vi "backup step.vi"(8 "error in (no error)":errorcluster, 10 "page":i32, 11 "backup_ref":u64) -> (0 "error out":errorcluster)   [LabVIEW 2020, in "sqlite3.lvlib"]
uses:
  sqlite3.lvlib
  errstr.vi
  bin/sqlite3_64.dll
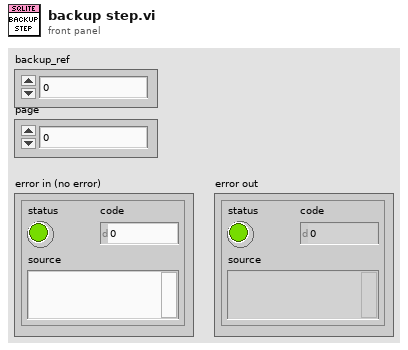
[diagram p1: front panel]
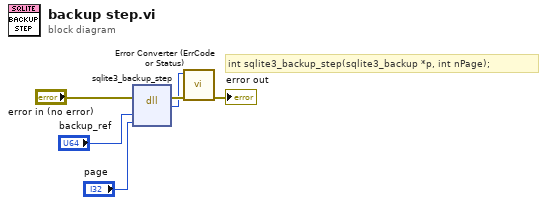
[diagram p0: block diagram]
diagram:
  # "int sqlite3_backup_step(sqlite3_backup *p, int nPage);"
  n1 = dll-call lib="D:/Project/Labview-Projects/database-configuration/externals/sqlite3/Source/bin/sqlite3_*.*" fn="sqlite3_backup_step"(error in="error in (no error)", "backup_ref"="backup_ref", "page"="page") -> (error out=w3:errorcluster, "return type"=w1:i32)  [unwired: 4 in, 1 out]
  n2 = call "Error Converter (ErrCode or Status).vi"("error in (no error)"=w3, "error code"=w1) -> ("error out"=→"error out":errorcluster)  [unwired: 9 in]
